vi "Max_Min_Measurement_Graph.vi"(1 "Graph Reference":refnum<vi>[](array[refnum]), 2 "Measurement Graphs (in)":T1[](array[typedef]) {"Y-Axis Array" items=["Time", "LI1CH1", "LI1CH2", "LI2CH1", "LI2CH2", "LI3CH1", "LI3CH2", "Field", "Temp", "Temp 2", "Temp 3", "N_Level", "H_Level", "Heat_370", "Sorb_Heat", "Still_Heat", "Capacity", "Loss", "Magnet_Temperature", "Lam_Pressure", "Lam_NValve", "370-T1", "370-T2", "370-T3", "370-T4", "370-T5", "370-R1", "370-R2", "370-R3", "370-R4", "370-R5", "372-T1", "372-T2", "372-T3", "372-T4", "372-T5", "372-T6", "372-R1", "372-R2", "372-R3", "372-R4", "372-R5", "372-R6", "Nada", "K2440_Res", "K2440_Current", "VTI_Heater", "VTI_NValve", "LS340_Heater", "K6221_Amplitude", "K6221_Frequency", "Cond_Pressure", "Still_Pressure", "FP_Out_Pressure", "Dump_Pressure", "V1", "V2", "V4", "V5", "V9", "Forepump", "Compressor", "K6221_Offset", "BoxTemp", "By", "Bz", "Phi", "heater-recond (%)", "Dewar Pressure ", "JT-SP-Control", "350 T1", "350 T2", "350 T3", "350 T4", "350 R1", "350 R2", "350 R3", "350 R4", "Angle"]; "X-Axis" items=["Time", "LI1CH1", "LI1CH2", "LI2CH1", "LI2CH2", "LI3CH1", "LI3CH2", "Field", "Temp", "Temp 2", "Temp 3", "N_Level", "H_Level", "Heat_370", "Sorb_Heat", "Still_Heat", "Capacity", "Loss", "Magnet_Temperature", "Lam_Pressure", "Lam_NValve", "370-T1", "370-T2", "370-T3", "370-T4", "370-T5", "370-R1", "370-R2", "370-R3", "370-R4", "370-R5", "372-T1", "372-T2", "372-T3", "372-T4", "372-T5", "372-T6", "372-R1", "372-R2", "372-R3", "372-R4", "372-R5", "372-R6", "Nada", "K2440_Res", "K2440_Current", "VTI_Heater", "VTI_NValve", "LS340_Heater", "K6221_Amplitude", "K6221_Frequency", "Cond_Pressure", "Still_Pressure", "FP_Out_Pressure", "Dump_Pressure", "V1", "V2", "V4", "V5", "V9", "Forepump", "Compressor", "K6221_Offset", "BoxTemp", "By", "Bz", "Phi", "heater-recond (%)", "Dewar Pressure ", "JT-SP-Control", "350 T1", "350 T2", "350 T3", "350 T4", "350 R1", "350 R2", "350 R3", "350 R4", "Angle"]}) -> (0 "Measurement Graphs (out)":T1[](array[typedef]) {"Y-Axis Array" items=["Time", "LI1CH1", "LI1CH2", "LI2CH1", "LI2CH2", "LI3CH1", "LI3CH2", "Field", "Temp", "Temp 2", "Temp 3", "N_Level", "H_Level", "Heat_370", "Sorb_Heat", "Still_Heat", "Capacity", "Loss", "Magnet_Temperature", "Lam_Pressure", "Lam_NValve", "370-T1", "370-T2", "370-T3", "370-T4", "370-T5", "370-R1", "370-R2", "370-R3", "370-R4", "370-R5", "372-T1", "372-T2", "372-T3", "372-T4", "372-T5", "372-T6", "372-R1", "372-R2", "372-R3", "372-R4", "372-R5", "372-R6", "Nada", "K2440_Res", "K2440_Current", "VTI_Heater", "VTI_NValve", "LS340_Heater", "K6221_Amplitude", "K6221_Frequency", "Cond_Pressure", "Still_Pressure", "FP_Out_Pressure", "Dump_Pressure", "V1", "V2", "V4", "V5", "V9", "Forepump", "Compressor", "K6221_Offset", "BoxTemp", "By", "Bz", "Phi", "heater-recond (%)", "Dewar Pressure ", "JT-SP-Control", "350 T1", "350 T2", "350 T3", "350 T4", "350 R1", "350 R2", "350 R3", "350 R4", "Angle"]; "X-Axis" items=["Time", "LI1CH1", "LI1CH2", "LI2CH1", "LI2CH2", "LI3CH1", "LI3CH2", "Field", "Temp", "Temp 2", "Temp 3", "N_Level", "H_Level", "Heat_370", "Sorb_Heat", "Still_Heat", "Capacity", "Loss", "Magnet_Temperature", "Lam_Pressure", "Lam_NValve", "370-T1", "370-T2", "370-T3", "370-T4", "370-T5", "370-R1", "370-R2", "370-R3", "370-R4", "370-R5", "372-T1", "372-T2", "372-T3", "372-T4", "372-T5", "372-T6", "372-R1", "372-R2", "372-R3", "372-R4", "372-R5", "372-R6", "Nada", "K2440_Res", "K2440_Current", "VTI_Heater", "VTI_NValve", "LS340_Heater", "K6221_Amplitude", "K6221_Frequency", "Cond_Pressure", "Still_Pressure", "FP_Out_Pressure", "Dump_Pressure", "V1", "V2", "V4", "V5", "V9", "Forepump", "Compressor", "K6221_Offset", "BoxTemp", "By", "Bz", "Phi", "heater-recond (%)", "Dewar Pressure ", "JT-SP-Control", "350 T1", "350 T2", "350 T3", "350 T4", "350 R1", "350 R2", "350 R3", "350 R4", "Angle"]})   [LabVIEW 2018]
uses:
  Plot.ctl
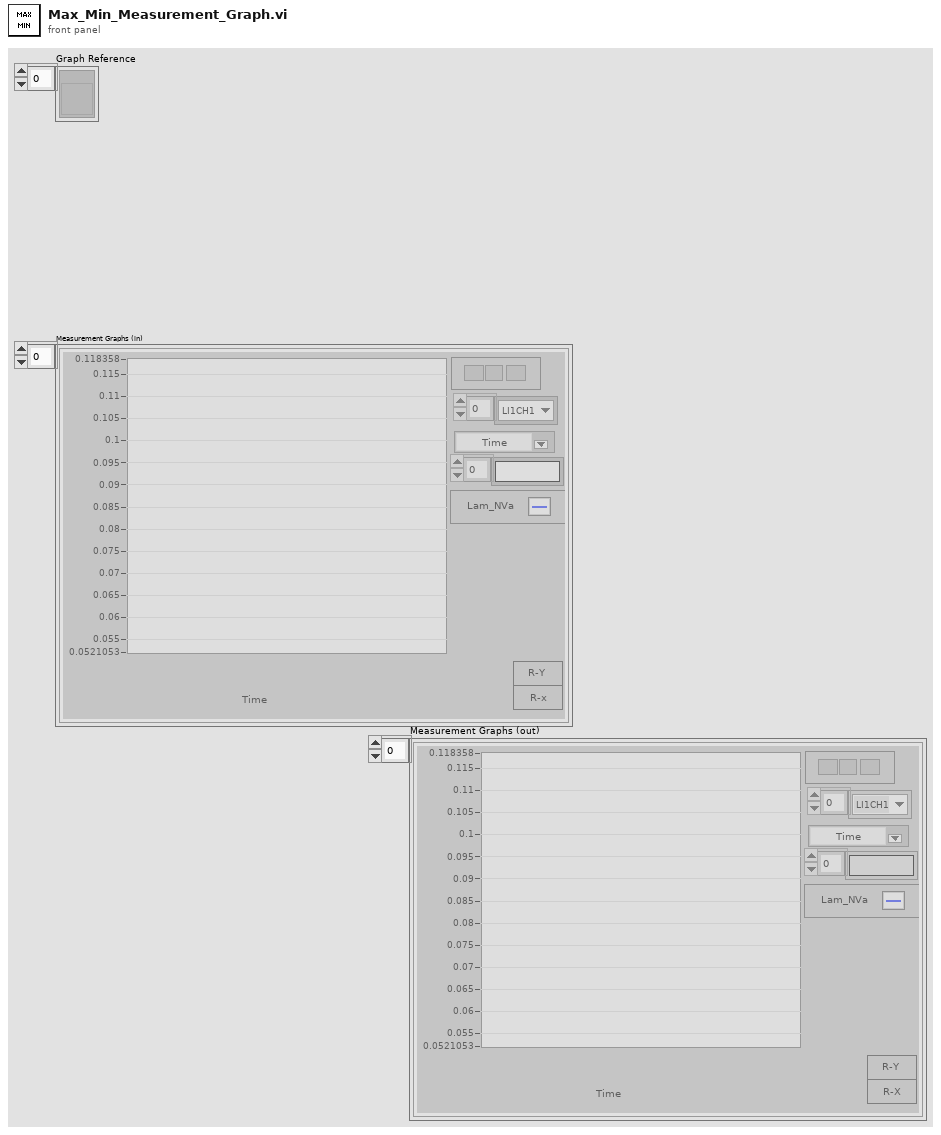
[diagram p1: front panel]
types:
  T1 = typedef "Plot.ctl" = cluster{"Measurement Graph":cluster{"Y":dbl[], "X":dbl[]}[], "X-Axis":i16, "Y-Axis Array":i16[], "Scale Plot":string[], "Rescale X":bool, "Rescale Y":bool}
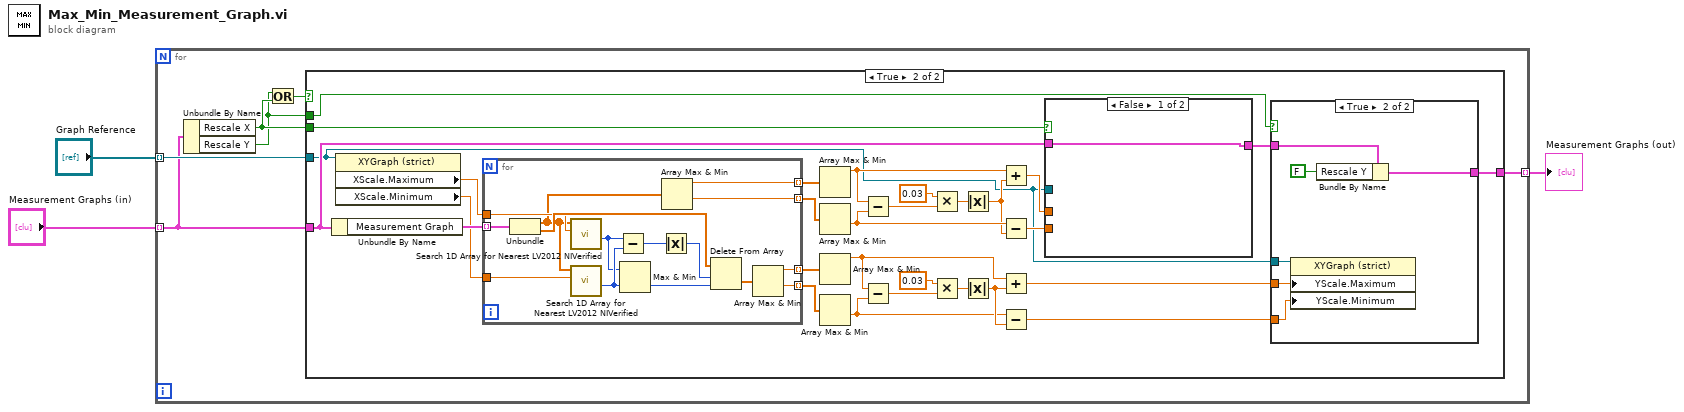
[diagram p0: block diagram]
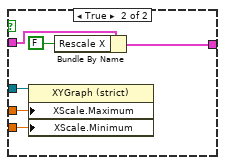
[diagram p4: hidden frame]
diagram:
  n1 = for {
    tunnel: "Graph Reference" -> [w9] mode=indexing
    tunnel: "Measurement Graphs (in)" -> [w4] mode=indexing
    tunnel: [w8] -> w1 mode=indexing
    n2 = Unbundle By Name(w4) -> ("Rescale X"=w6:bool, "Rescale Y"=w5:bool)
    n3 = Or(x=w5, y=w6) -> (x .or. y?=w7:bool)
    n4 = case shown="True" w7 {
      tunnel: w9 -> [_ w21]
      tunnel: w4 -> [w10 w35]
      tunnel: [w10 w38] -> w8
      tunnel: w6 -> [_ w37]
      tunnel: w5 -> [_ w36]
      frame False {
      }
      frame True {
        n5 = Unbundle By Name(w35) -> ("Measurement Graph"=w30:cluster{"Y":dbl[], "X":dbl[]}[])
        n6 = property on="Property Node" class="XYGraph (strict)"(reference=w21) -> ("XScale.Maximum"=w19:dbl, "XScale.Minimum"=w20:dbl)  [unwired: 1 in, 2 out]
        n7 = for {
          tunnel: w30 -> [w54] mode=indexing
          tunnel: [w51] -> w34 mode=indexing
          tunnel: [w50] -> w33 mode=indexing
          tunnel: [w53] -> w32 mode=indexing
          tunnel: [w52] -> w31 mode=indexing
          tunnel: w20 -> [w42]
          tunnel: w19 -> [w44]
          n8 = Unbundle(w54) -> ("Y"=w43:dbl[], "X"=w47:dbl[])
          n9 = call "Search 1D Array for Nearest LV2012 NIVerified.vi"("desired element"=w44, "1D Array"=w43) -> ("closest index"=w40:i32)  [unwired: 8 in, 1 out]
          n10 = call "Search 1D Array for Nearest LV2012 NIVerified.vi"("desired element"=w42, "1D Array"=w43) -> ("closest index"=w41:i32)  [unwired: 8 in, 1 out]
          n11 = Subtract(x=w40, y=w41) -> (x-y=w46:i32)
          n12 = Max & Min(x=w40, y=w41) -> (min(x,y)=w49:i32)  [unwired: 1 out]
          n13 = Absolute Value(x=w46) -> (abs(x)=w45:i32)
          n14 = Array Max & Min(array=w43) -> (max value=w50:dbl, min value=w51:dbl)  [unwired: 2 out]
          n15 = Delete From Array(array=w47, length=w45, index=w49) -> (deleted portion=w48:dbl[])  [unwired: 1 out]
          n16 = Array Max & Min(array=w48) -> (max value=w53:dbl, min value=w52:dbl)  [unwired: 2 out]
        }
        n17 = Array Max & Min(array=w33) -> (max value=w25:dbl)  [unwired: 3 out]
        n18 = Array Max & Min(array=w34) -> (min value=w24:dbl)  [unwired: 3 out]
        n19 = Array Max & Min(array=w32) -> (max value=w11:dbl)  [unwired: 3 out]
        n20 = Array Max & Min(array=w31) -> (min value=w14:dbl)  [unwired: 3 out]
        n21 = Subtract(x=w25, y=w24) -> (x-y=w28:dbl)
        n22 = Subtract(x=w11, y=w14) -> (x-y=w17:dbl)
        n23 = Multiply(x=0.03, y=w28) -> (x*y=w23:dbl)
        n24 = Multiply(x=0.03, y=w17) -> (x*y=w16:dbl)
        n25 = Absolute Value(x=w23) -> (abs(x)=w22:dbl)
        n26 = Absolute Value(x=w16) -> (abs(x)=w15:dbl)
        n27 = Add(x=w25, y=w22) -> (x+y=w26:dbl)
        n28 = Subtract(x=w24, y=w22) -> (x-y=w27:dbl)
        n29 = Add(x=w11, y=w15) -> (x+y=w12:dbl)
        n30 = Subtract(x=w14, y=w15) -> (x-y=w13:dbl)
        n31 = case shown="False" w37 {
          tunnel: w21 -> [_ w68]
          tunnel: w26 -> [_ w67]
          tunnel: w27 -> [_ w63]
          tunnel: w35 -> [w62 w66]
          tunnel: [w62 w64] -> w39
          frame False {
          }
          frame True {
            n32 = property on="Property Node" class="XYGraph (strict)"(reference=w68, "XScale.Maximum"=w67, "XScale.Minimum"=w63) -> ()  [unwired: 1 in, 2 out]
            n33 = Bundle By Name(cluster=w66, "Rescale X"=FALSE) -> (w64:T1)
          }
        }
        n34 = case shown="True" w36 {
          tunnel: w39 -> [w55 w61]
          tunnel: [w55 w60] -> w38
          tunnel: w13 -> [_ w58]
          tunnel: w21 -> [_ w57]
          tunnel: w12 -> [_ w56]
          frame False {
          }
          frame True {
            n35 = property on="Property Node" class="XYGraph (strict)"(reference=w57, "YScale.Maximum"=w56, "YScale.Minimum"=w58) -> ()  [unwired: 1 in, 2 out]
            n36 = Bundle By Name(cluster=w61, "Rescale Y"=FALSE) -> (w60:T1)
          }
        }
      }
    }
  }
  "Measurement Graphs (out)" <- w1
